vi "DAQmx terminal Name.vi"(1 "DAQmx Terminal Name":tag) -> (0 "DAQmx Terminal Name Out":tag)   [LabVIEW 2013]
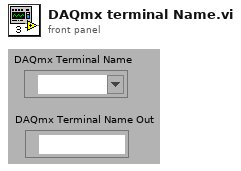
[diagram p1: front panel]
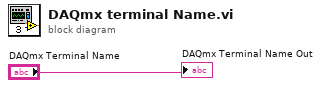
[diagram p0: block diagram]
diagram:
  "DAQmx Terminal Name Out" <- "DAQmx Terminal Name"
